vi "Display.vi"(8 "error in":errorcluster, 11 "One Button in":refnum<class "One Button.lvclass">) -> (0 "error out":errorcluster, 3 "One Button out":refnum<class "One Button.lvclass">)   [LabVIEW 2021, in "Pop-Up.lvlib" / "One Button.lvclass"]
doc: "This vi will display the one button popup with the supplied graphic and text label (contained in the object). It will wait for a button press.\n\n<b>Code Developed By:</b>\nDaniel Coons\nTechnology Service Corporation\n1983 S Liberty Drive\nBloomington, IN 47403\nPhone: 812 558-7100\ndaniel.coons@tsc.com\nwww.tsc.com/atcs"
uses:
  One Button.lvclass
  C:/Development/Open Source/tsc-pop-up/Popup/Popup.lvclass
  Popup/Popup.lvclass/Popup.ctl
  Popup/Data Member Access/Read Theme.vi
  Theme/Theme.lvclass
  Popup/Popup.lvclass
  user32.dll
panel:
  out "header":bool
  in  "OK Button":bool
  out "2D Picture":picture
  out "message":string
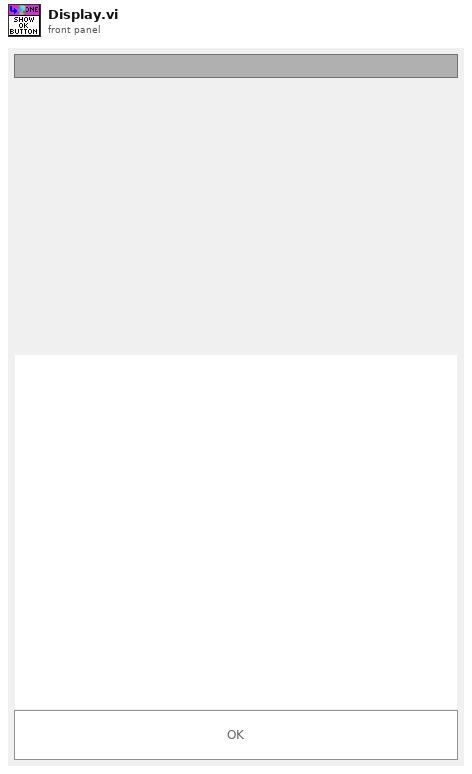
[diagram p1: front panel]
types:
  T1 = typedef "LVPoint32TypeDef.ctl" = cluster{"Horizontal":i32, "Vertical":i32}
  T2 = typedef "LVPositionTypeDef.ctl" = cluster{"Left":i32, "Top":i32}
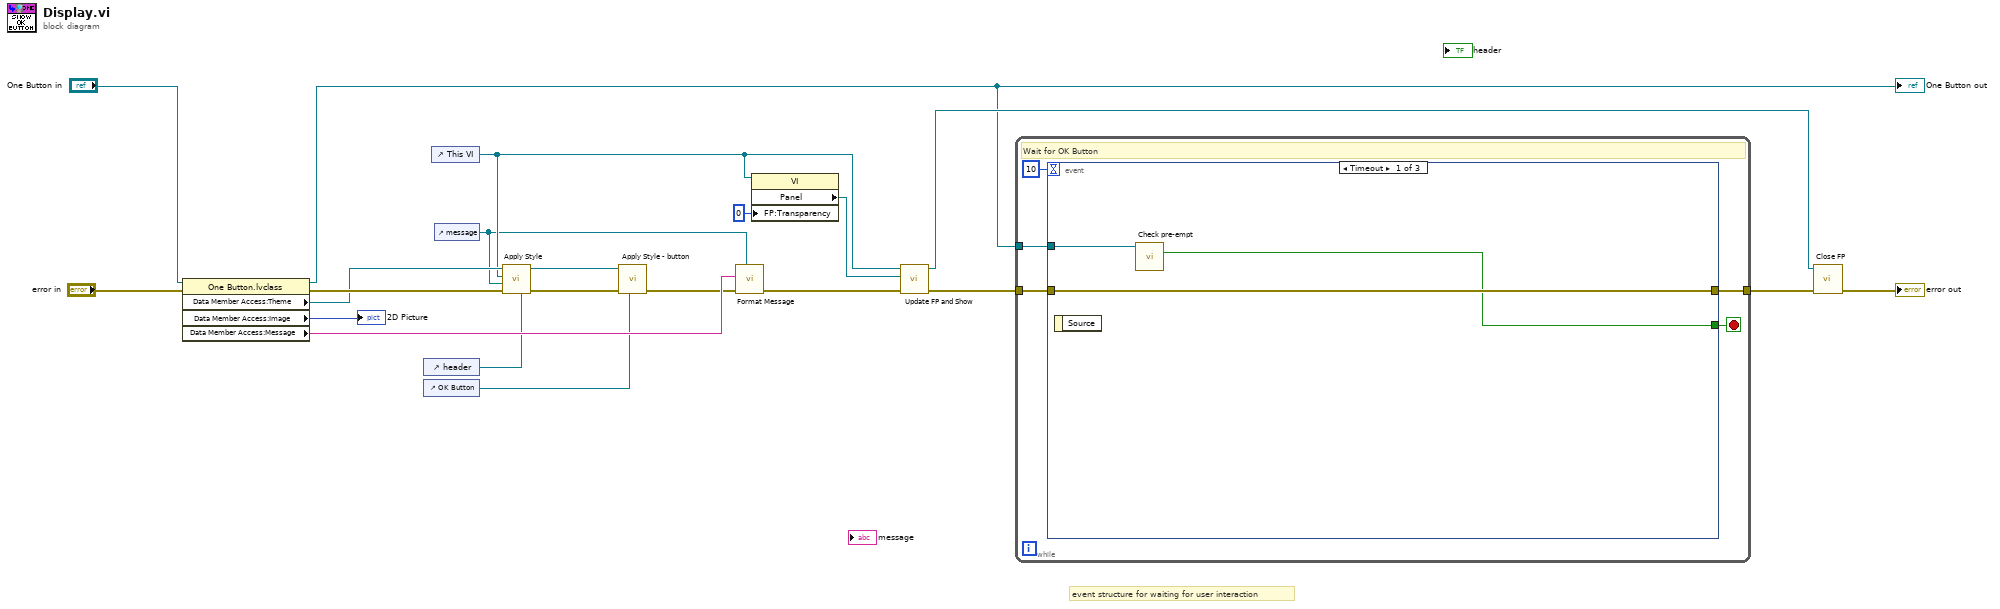
[diagram p0: block diagram]
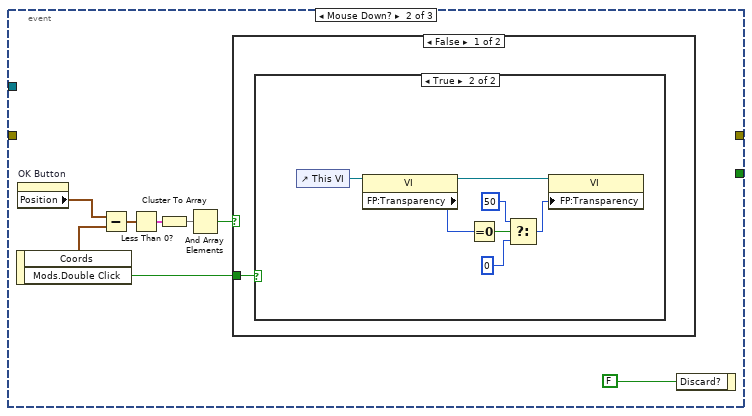
[diagram p2: hidden frame]
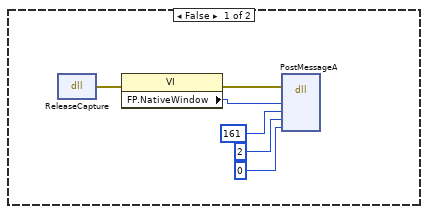
[diagram p3: hidden frame]
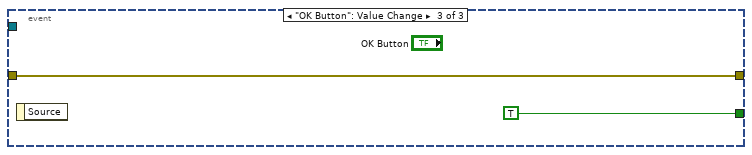
[diagram p5: hidden frame]
diagram:
  # "event structure for waiting for user interaction"
  n1 = property class="One Button.lvclass"(reference="One Button in", error in="error in") -> (reference out=w12:refnum<class "One Button.lvclass">, error out=w20:errorcluster, "Data Member Access:Theme"=w8:refnum<class "Theme.lvclass">, "Data Member Access:Image"=→"2D Picture":picture, "Data Member Access:Message"=w11:string)
  "One Button out" <- w12
  n2 = control-ref of="header"() -> (w5:refnum<vi>)
  n3 = control-ref of="OK Button"() -> (w2:refnum<vi>)
  n4 = control-ref of="This VI"() -> (w7:refnum<vi>)
  n5 = control-ref of="message"() -> (w6:refnum<vi>)
  n6 = call "Apply Style.vi"("header ref"=w5, "error in"=w20, "message ref"=w6, "pop up ref"=w7, "Theme in"=w8) -> ("error out"=w9:errorcluster, "Theme out"=w3:refnum<class "Theme.lvclass">)  [unwired: 5 in]
  n7 = call "Apply Style - button.vi"("button ref"=w2, "error in"=w9, "Theme in"=w3) -> ("error out"=w4:errorcluster)  [unwired: 7 in, 1 out]
  n8 = call "Format Message.vi"("formatted string"=w6, "error in"=w4, "String Input"=w11) -> ("error out"=w10:errorcluster)  [unwired: 7 in, 1 out]
  n9 = property class="VI"(reference=w7, "FP:Transparency"=u8 0 ("Front Panel Window:Transparency")) -> ("Panel"=w16:refnum<vi>)  [unwired: 1 in, 2 out]
  n10 = call "Update FP and Show.vi"("error in (no error)"=w10, "Panel Ref"=w16, "VI in"=w7) -> ("error out"=w15:errorcluster, "VI out"=w13:refnum<vi>)  [unwired: 7 in]
  n11 = while {
    tunnel: [w24] -> w17
    tunnel: w15 -> [w25]
    tunnel: w12 -> [w22]
    stop <- w26 stop-if-true
    # "Wait for OK Button"
    n12 = event shown="[0] Timeout" {
      selector: _ -> [_ _ _]
      dyn-events: _ -> [_ _ _]
      timeout: 10 -> [_ _ _]
      tunnel: [w27 _ TRUE ("OK Button")] -> w26
      tunnel: w25 -> [w29 _ w52]
      tunnel: [w29 _ w52] -> w24
      tunnel: w22 -> [w28 _ _]
      event Timeout {
        n13 = event-data() -> ()  [unwired: 1 in, 1 out]
        n14 = call "Check pre-empt.vi"("_Popup in"=w28) -> ("Pre-empted?"=w27:bool)  [unwired: 8 in, 2 out]
      }
      event Mouse Down? {
        n15 = event-data() -> ("Coords"=w36:T1, "Mods.Double Click"=w30:bool)  [unwired: 1 in]
        n16 = property on="OK Button" class="Bool"() -> ("Position"=w35:T2)  [unwired: 2 in, 2 out]
        n17 = Subtract(x=w35, y=w36) -> (x-y=w34:T2)
        n18 = Less Than 0?(x=w34) -> (x < 0?=w33:cluster{"Left":bool, "Top":bool})
        n19 = Cluster To Array(cluster=w33) -> (array=w32:bool[])
        n20 = And Array Elements(Boolean array=w32) -> (logical AND=w31:bool)
        n21 = case shown="False" w31 {
          tunnel: w30 -> [w38 _]
          frame False {
            n22 = case shown="True" w38 {
              frame False {
                n23 = dll-call lib="user32.dll" fn="ReleaseCapture"() -> (error out=w42:errorcluster)  [unwired: 4 in, 1 out]
                n24 = property class="VI"(error in=w42) -> (error out=w43:errorcluster, "FP.NativeWindow"=w44:u64)  [unwired: 1 in, 1 out]
                n25 = dll-call lib="user32.dll" fn="PostMessageA"(error in=w43, "hWnd"=w44, "Msg"=161, "wParam"=2, "lParam"=0) -> ()  [unwired: 7 in, 2 out]
              }
              frame True {
                n26 = control-ref of="This VI"() -> (w51:refnum<vi>)
                n27 = property class="VI"(reference=w51) -> (reference out=w49:refnum<vi>, "FP:Transparency"=w50:u8)  [unwired: 1 in, 1 out]
                n28 = Equal To 0?(x=w50) -> (x = 0?=w48:bool)
                n29 = Select(t=u8 50, s=w48, f=u8 0) -> (s? t:f=w47:u8)
                n30 = property class="VI"(reference=w49, "FP:Transparency"=w47) -> ()  [unwired: 1 in, 2 out]
              }
            }
          }
          frame True {
          }
        }
        n31 = event-data("Discard?"=FALSE) -> ()  [unwired: 1 in, 1 out]
      }
      event "OK Button": Value Change {
        n32 = event-data() -> ()  [unwired: 1 in, 1 out]
      }
    }
  }
  n33 = call "Close FP.vi"("error in (no error)"=w17, "VI in"=w13) -> ("error out"=→"error out":errorcluster)  [unwired: 9 in]
